vi "loadAmicHistData.vi"() -> ()   [LabVIEW 2012]
uses:
  <vilib>/Utility/file.llb/Read From Spreadsheet File (string).vi
panel:
  out "element 2":string
  out "error out 2":errorcluster
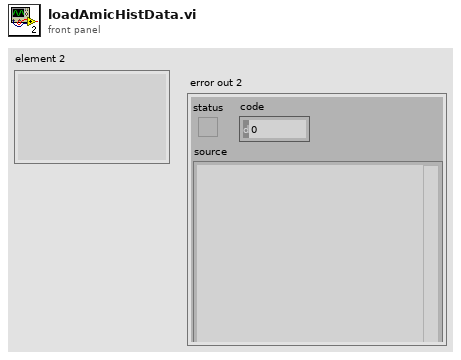
[diagram p1: front panel]
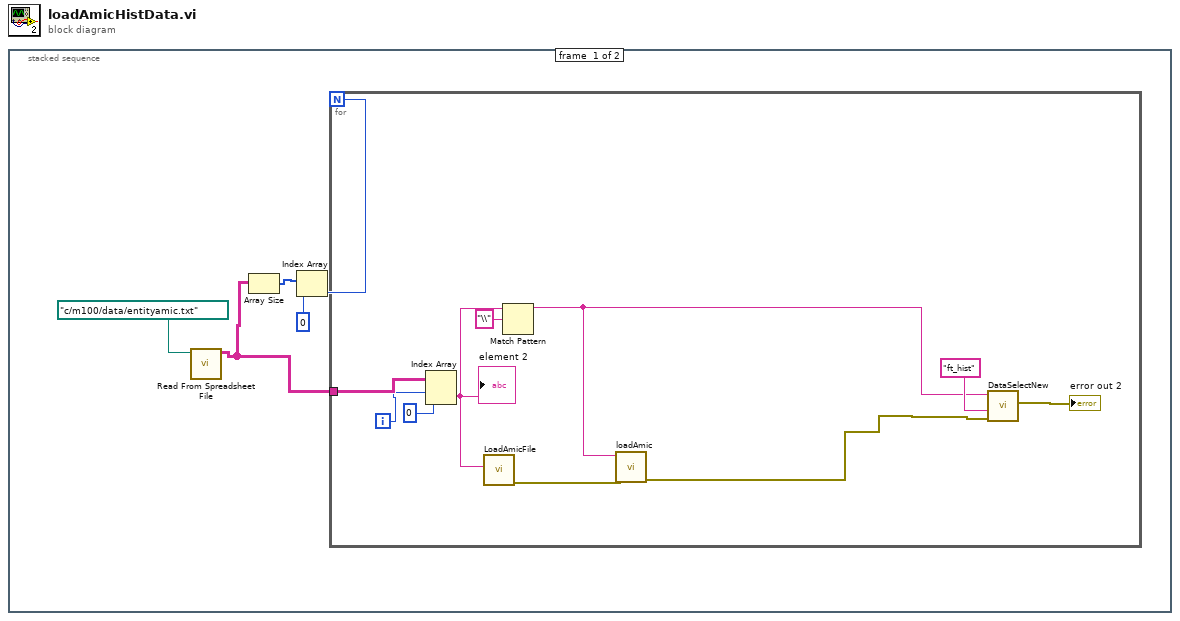
[diagram p0: block diagram]
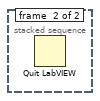
[diagram p2: hidden frame]
diagram:
  n1 = stacked-sequence {
    frame #0 {
      n2 = call-poly <vilib>:"Read From Spreadsheet File.vi"("file path (dialog if empty)"=path "c:/m100/data/entityamic.txt" ("file path (use dialog)")) -> ("all rows"=w1:string[][])  [unwired: 6 in, 4 out]
      n3 = Array Size(array=w1) -> (size(s)=w4:i32[])
      n4 = Index Array(array=w4, index=0) -> (element=w2:i32)
      n5 = for {
        N: w2 -> [_]
        tunnel: w1 -> [w15]
        i -> [w13]
        n6 = Index Array(array=w15, index (row)=w13, index (col)=0 ("disabled index (col)")) -> (element=w9:string)
        "element 2" <- w9
        n7 = call "LoadAmicFile.vi"("folder"=w9) -> ("error out"=w8:errorcluster)  [unwired: 9 in, 1 out]
        n8 = Match Pattern(string=w9, regular expression="\\") -> (before substring=w7:string)  [unwired: 1 in, 3 out]
        n9 = call "loadAmic.vi"("error in"=w8, "machine"=w7) -> ("error out"=w6:errorcluster)  [unwired: 9 in]
        n10 = call "DataSelectNew.vi"("error in (no error)"=w6, "Table"="ft_hist", "Machine"=w7) -> ("error out"=→"error out 2":errorcluster)  [unwired: 8 in]
      }
    }
    frame #1 {
      n11 = Quit LabVIEW() -> ()  [unwired: 1 in]
    }
  }
